vi "PQexpressCmd.vi"(8 "error in (no error)":errorcluster, 10 "Command":string, 11 "conninfo":T1={"host"="localhost", "port"="5432", "client_encoding"="UTF8", "dbname"="data", "user"="postgres", "password"=""}) -> (0 "error out":errorcluster, 1 "DatabaseMessages":T2, 2 "column_names":string[](array[string]), 3 "data":string[][](array[string]))   [LabVIEW 2019, in "libpqutility64.lvlib"]
doc: "set the connection string, type in your SQL cmd and fire! The Result Data is provided as Array of String"
uses:
  libpqutility64.lvlib
  libpqlv64/src/PQfinish.vi
  libpqlv64/src/PQconnectdb.vi
  libpqlv64/src/PQerrorMessage.vi
  libpqlv64/src/PQstatus.vi
  <vilib>/dlg_ctls.llb/Space Constant.vi
  libpqlv64/src/PQclear.vi
  PQsyncQueryCommand.vi
  PQfetchResultData.vi
  PQfetchColumnNames.vi
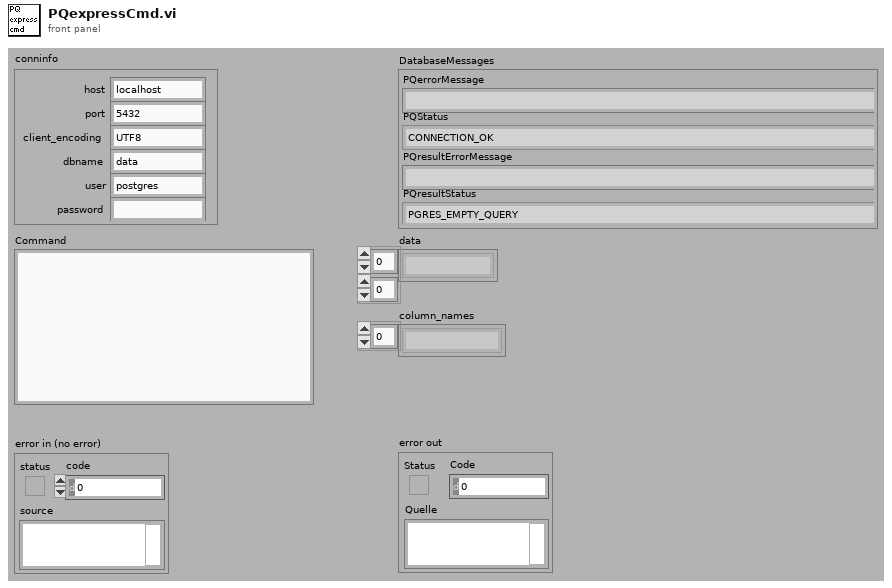
[diagram p1: front panel]
types:
  T1 = cluster{"host":string, "port":string, "client_encoding":string, "dbname":string, "user":string, "password":string}
  T2 = cluster{"PQerrorMessage":string, "PQStatus":enum16{"CONNECTION_OK", "CONNECTION_BAD", "CONNECTION_STARTED", "CONNECTION_MADE", "CONNECTION_AWAITING_RESPONSE", "CONNECTION_AUTH_OK", "CONNECTION_SETENV", "CONNECTION_SSL_STARTUP", "CONNECTION_NEEDED"}, "PQresultErrorMessage":string, "PQresultStatus":enum16{"PGRES_EMPTY_QUERY", "PGRES_COMMAND_OK", "PGRES_TUPLES_OK", "PGRES_COPY_OUT", "PGRES_COPY_IN", "PGRES_BAD_RESPONSE", "PGRES_NONFATAL_ERROR", "PGRES_FATAL_ERROR"}}
  T3 = enum32{"CONNECTION_OK", "CONNECTION_BAD", "CONNECTION_STARTED", "CONNECTION_MADE", "CONNECTION_AWAITING_RESPONSE", "CONNECTION_AUTH_OK", "CONNECTION_SETENV", "CONNECTION_SSL_STARTUP", "CONNECTION_NEEDED"}
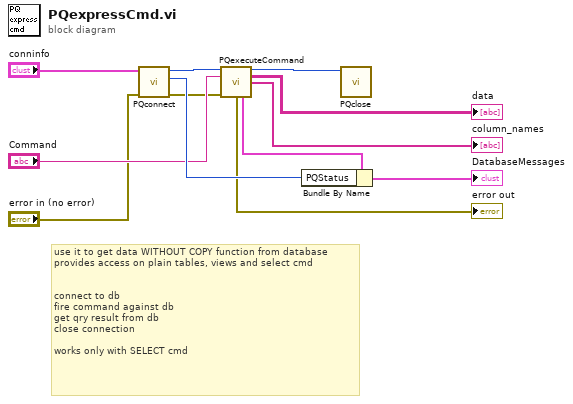
[diagram p0: block diagram]
diagram:
  # "use it to get data WITHOUT COPY function from database\nprovides access on plain tables, views and select cmd\n\n\nconnect to db\nfire command against db\nget qry result from db\nclose connection\n\nworks only with SELECT cmd"
  n1 = call "PQconnect.vi"("error in (no error)"="error in (no error)", "conninfo"="conninfo") -> ("error out"=w1:errorcluster, "PQStatus"=w12:T3, "conn"=w10:u64)  [unwired: 7 in]
  n2 = call "PQexecuteCommand.vi"("conn"=w10, "Command"="Command", "error in (no error)"=w1) -> ("conn_out"=w8:u64, "Data"=→"data":string[][], "ColumnNames"=→"column_names":string[], "error out"=→"error out":errorcluster, "DatabaseMesssageCluster"=w5:T2)  [unwired: 6 in, 2 out]
  n3 = Bundle By Name(cluster=w5, "PQStatus"=w12) -> (→"DatabaseMessages":T2)
  n4 = call "PQclose.vi"("conn"=w8) -> ()  [unwired: 10 in, 1 out]
